vi "Expand Contract Status Pane.vi"(7 "Action":enum16{"Init", "Expand", "Contract"}(ring), 8 "Error In":errorcluster, 11 "Status Splitter":refnum<vi>) -> (0 "Error Out":errorcluster)   [LabVIEW 2014]
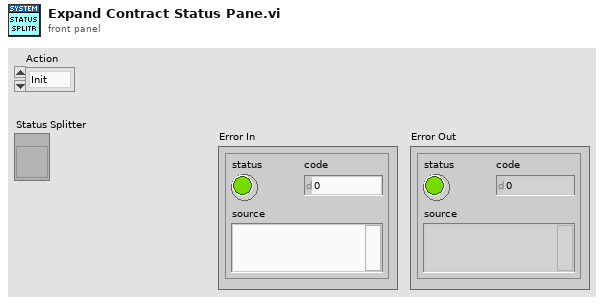
[diagram p1: front panel]
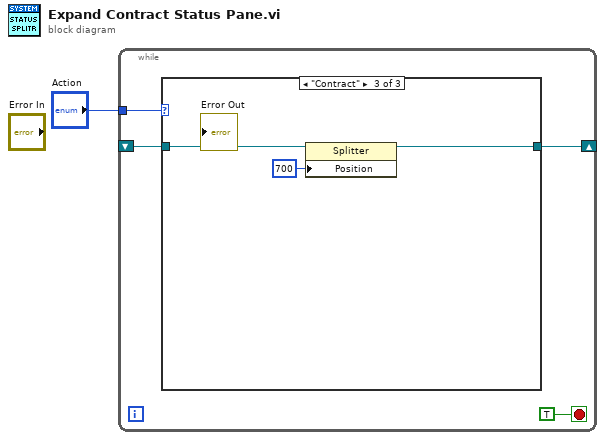
[diagram p0: block diagram]
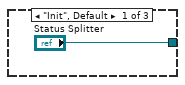
[diagram p2: hidden frame]
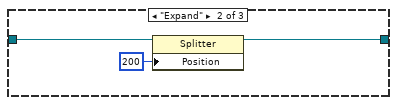
[diagram p3: hidden frame]
diagram:
  n1 = while {
    tunnel: "Action" -> [w5]
    shift-right: [w3] -> _
    shift-left: _ -> [w2]
    stop <- TRUE stop-if-true
    n2 = case shown="\"Contract\"" w5 {
      tunnel: ["Status Splitter" w8 w11] -> w3
      tunnel: w2 -> [_ w9 w12]
      frame "Init", Default {
      }
      frame "Expand" {
        n3 = property class="Splitter"(reference=w9, "Position"=200 ("Splitter Position")) -> (reference out=w8:refnum<vi>)  [unwired: 1 in, 1 out]
      }
      frame "Contract" {
        n4 = property class="Splitter"(reference=w12, "Position"=700 ("Splitter Position")) -> (reference out=w11:refnum<vi>)  [unwired: 1 in, 1 out]
      }
    }
  }
